vi "EX 2-3 Fade_port.vi"() -> ()   [LabVIEW 2011]
uses:
  <vilib>/LabVIEW Interface for Arduino/Type Defs/Board Type.ctl
  <vilib>/LabVIEW Interface for Arduino/Type Defs/Connection Type.ctl
  <vilib>/LabVIEW Interface for Arduino/LabVIEW Interface for Arduino.lvlib
panel:
  in  "Knob":u16(knob) scale=0.0..255.0
  out "PWM":i32
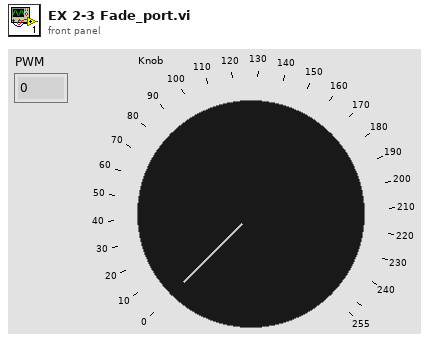
[diagram p1: front panel]
types:
  T1 = typedef "LabVIEW Interface for Arduino.lvlib/Connection Type.ctl" = enum8{"USB / Serial", "XBEE", "BlueSmirf (Bluetooth)"}
  T2 = typedef "LabVIEW Interface for Arduino.lvlib/Board Type.ctl" = enum16{"Uno", "Dimuelanove w/Atmega 328", "Mega 2560"}
  T3 = typedef "LabVIEW Interface for Arduino.lvlib/Arduino Resource.ctl" = cluster{"VISA resource":refnum<visa-resource-name>, "Board Type":T2, "Connection Type":enum8{"USB / Serial"}, "Bytes Per Packet (15)":u8}
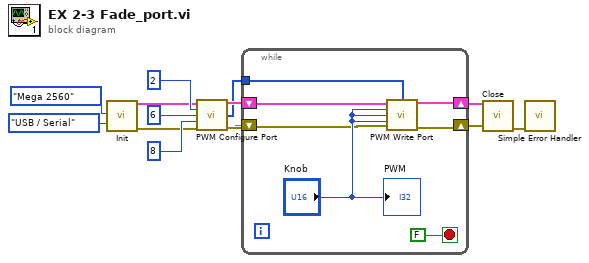
[diagram p0: block diagram]
diagram:
  n1 = call <vilib>:"Init.vi"("Board Type (Uno)"=Board_Type."Mega 2560", "Connection Type (USB/Serial)"=Connection_Type."USB / Serial") -> ("Arduino Resource"=w3:T3, "error out"=w2:errorcluster)  [unwired: 16 in]
  n2 = call <vilib>:"PWM Configure Port.vi"("Arduino Resource"=w3, "PWM Pin (3)"=u8 2 ("Digital I/O Pin"), "PWM Pin (5)"=u8 6 ("Digital I/O Pin"), "PWM Pin (6)"=u8 8 ("Digital I/O Pin"), "error in"=w2) -> ("Arduino Resource"=w5:T3, "PWM Pins"=w1:u8[], "error out"=w4:errorcluster)  [unwired: 8 in]
  n3 = while {
    shift-right: [w18] -> w13
    shift-left: w5 -> [w16]
    shift-right: [w19] -> w12
    shift-left: w4 -> [w15]
    tunnel: w1 -> [w14]
    stop <- FALSE stop-if-true
    n4 = call <vilib>:"PWM Write Port.vi"("Arduino Resource"=w16, "PWM Pins"=w14, "PWM 0 (0-255)"="Knob", "PWM 1 (0-255)"="Knob", "PWM 2 (0-255)"="Knob", "error in"=w15) -> ("Arduino Resource"=w18:T3, "error out"=w19:errorcluster)  [unwired: 7 in, 1 out]
    "PWM" <- "Knob"
  }
  n5 = call <vilib>:"Close.vi"("Arduino Resource"=w13, "error in"=w12) -> ("error out"=w11:errorcluster)  [unwired: 13 in]
  n6 = call <vilib>:"Simple Error Handler.vi"("error in (no error)"=w11) -> ()  [unwired: 4 in, 5 out]
